vi "Coord window-Add to picture-Motor coord.vi"(7 "Feature to draw":enum16{"Draw point", "Draw square"}(ring), 9 "Motor coordinates":cluster{"X":sgl, "Y":sgl, "Z":sgl}, 10 "new picture in":picture, 11 "Picture in":refnum<vi>) -> (2 "new picture":picture, 3 "Picture out":refnum<vi>)   [LabVIEW 2013]
uses:
  Globals/Coord window-Globals.vi
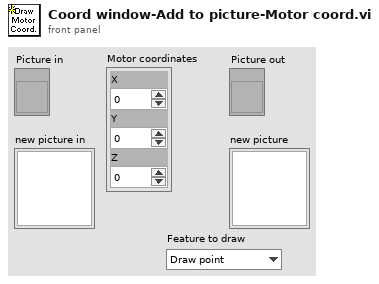
[diagram p1: front panel]
types:
  T1 = cluster{"Width":u16, "Style":enum32{"Solid", "Dash", "Dot", "DashDot", "DashDotDot"}}
  T2 = cluster{"left":i16, "top":i16, "right":i16, "bottom":i16}
  T3 = cluster{"Width":i16, "Style":enum32{"Solid", "Dash", "Dot", "DashDot", "DashDotDot"}}
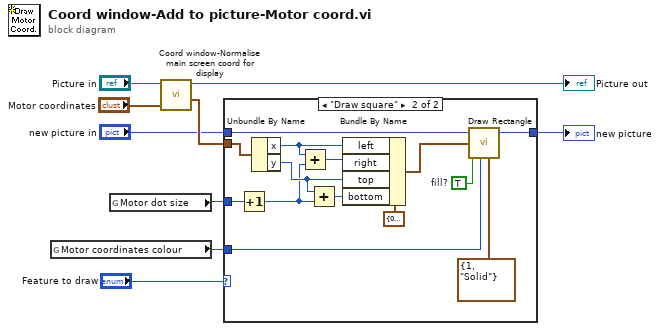
[diagram p0: block diagram]
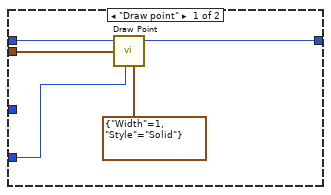
[diagram p2: hidden frame]
diagram:
  n1 = global read "Coord window-Globals.vi" "Motor coordinates colour"() -> (w2:u32)
  n2 = global read "Coord window-Globals.vi" "Motor dot size"() -> (w1:i16)
  n3 = call "Coord window-Normalise main screen coord for display.vi"("Motor coordinates"="Motor coordinates", "Picture map ref in"="Picture in") -> ("Normalised top level screen coordinates (for display)"=w5:cluster{"x":i16, "y":i16}, "Picture map ref"=→"Picture out":refnum<vi>)  [unwired: 8 in]
  n4 = case shown="\"Draw square\"" "Feature to draw" {
    tunnel: "new picture in" -> [w14 w28]
    tunnel: [w12 w27] -> w3
    tunnel: w5 -> [w11 w23]
    tunnel: w2 -> [w10 w26]
    tunnel: w1 -> [_ w16]
    frame "Draw point" {
      n5 = call <vilib>:"Draw Point.vi"("picture"=w14, "point(x,y)"=w11, "color(black)"=w10, "pen"=T1 {"Width"=1, "Style"=enum."Solid"}) -> ("new picture"=w12:picture)  [unwired: 5 in]
    }
    frame "Draw square" {
      w24 = TRUE  # fill?
      n6 = Increment(x=w16) -> (x+1=w15:i16)
      n7 = Unbundle By Name(w23) -> ("x"=w20:i16, "y"=w17:i16)
      n8 = Add(x=w20, y=w15) -> (x+y=w19:i16)
      n9 = Add(x=w17, y=w15) -> (x+y=w18:i16)
      n10 = Bundle By Name(cluster=T2 {"left"=0, "top"=0, "right"=0, "bottom"=0} ("rect"), "left"=w20, "right"=w19, "top"=w17, "bottom"=w18) -> (w21:T2)
      n11 = call <vilib>:"Draw Rectangle.vi"("picture"=w28, "rect"=w21, "fill?(F)"=w24, "color(black)"=w26, "pen"=T3 {"Width"=1, "Style"=enum."Solid"}) -> ("new picture"=w27:picture)  [unwired: 4 in]
    }
  }
  "new picture" <- w3
